vi "write TBM configuration.vi"(8 "error in":errorcluster, 10 "TBM configuration in":refnum<class "TBM configuration.lvclass">, 11 "Shared Library Module editor node in":refnum<class "Shared Library Module editor node.lvclass">) -> (0 "error out":errorcluster, 3 "Shared Library Module editor node out":refnum<class "Shared Library Module editor node.lvclass">)   [LabVIEW 2013, in "Shared Library Module editor node.lvclass"]
doc: "Platypus Framework 1.0.1.60\nNI Systems Engineering - National Instruments"
uses:
  Shared Library Module editor node.lvclass
  <vilib>/NI/Tag Bus Module Framework/root configuration/TBM configuration.lvclass
  <vilib>/TBM Modules/CLFN/configuration/Shared Library Module configuration.lvclass
  Shared Library Module editor node.lvclass/Shared Library Module editor node.ctl
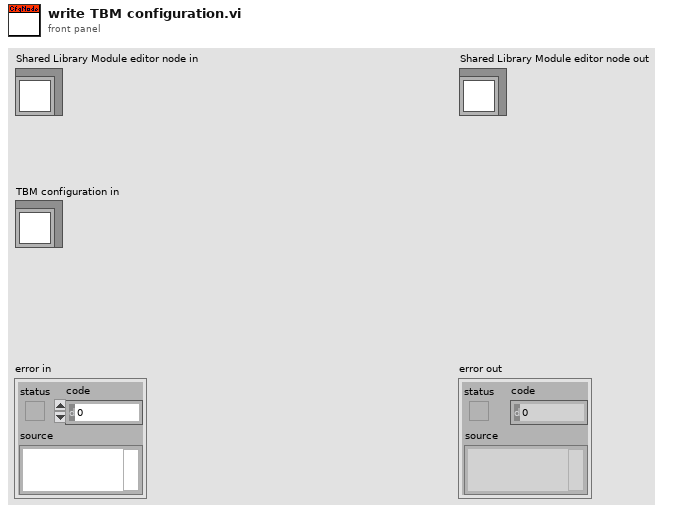
[diagram p1: front panel]
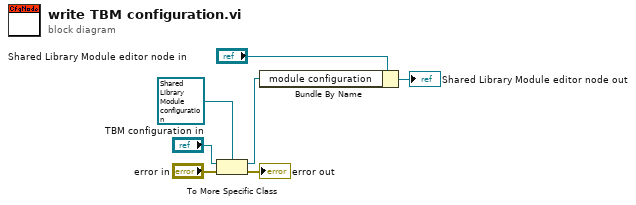
[diagram p0: block diagram]
diagram:
  n1 = To More Specific Class(target class=refnum<class "Shared Library Module configuration.lvclass"> refnum ("module configuration"), reference="TBM configuration in", error in="error in") -> (specific class reference=w1:refnum<class "Shared Library Module configuration.lvclass">, error out=→"error out":errorcluster)
  n2 = Bundle By Name(cluster="Shared Library Module editor node in", "module configuration"=w1) -> (→"Shared Library Module editor node out":refnum<class "Shared Library Module editor node.lvclass">)
